vi "pop_growth_A.vi"(8 "sat pol in":dbl, 10 "rho - val in":dbl, 11 "rho+ val in":dbl) -> (3 "Growth val out":dbl)   [LabVIEW 2018]
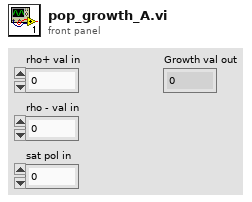
[diagram p1: front panel]
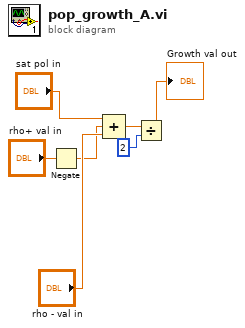
[diagram p0: block diagram]
diagram:
  n1 = Negate(x="rho+ val in") -> (-x=w4:dbl)
  n2 = Compound Arithmetic op=ADD("sat pol in", w4, "rho - val in") -> (w3:dbl)
  n3 = Divide(x=w3, y=2) -> (x/y=→"Growth val out":dbl)
